vi "Read.vi"() -> ()   [LabVIEW 2013]
uses:
  <vilib>/NI/Modbus Library/API/Master/Modbus Master.lvclass
  <vilib>/NI/Modbus Library/API/Wrapper/Create TCP Master.vi
  GlobalStop.vi
  GlobalGraph.vi
  <vilib>/NI/Modbus Library/API/Wrapper/API Main.lvlib
panel:
  out "error out":errorcluster
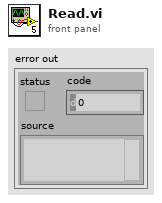
[diagram p1: front panel]
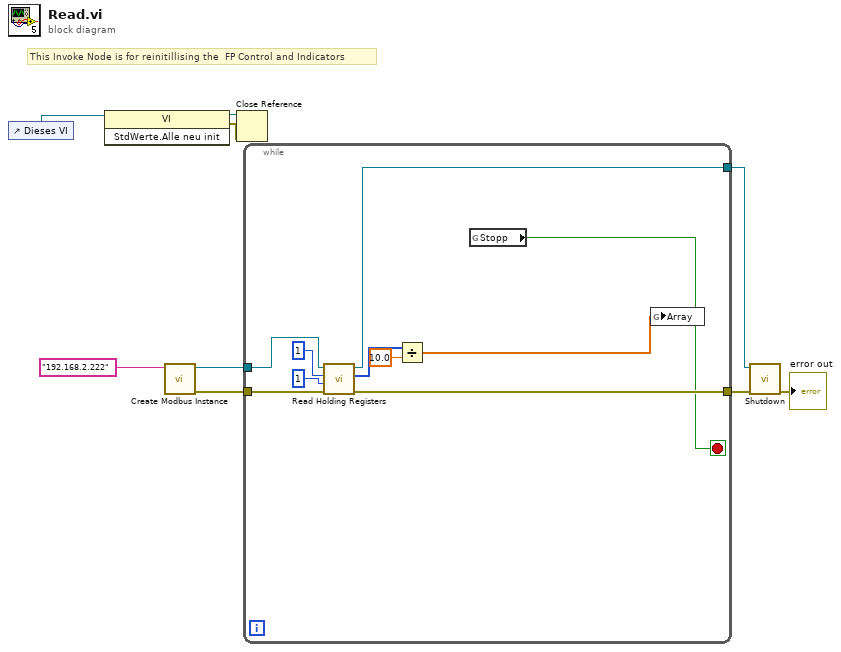
[diagram p0: block diagram]
diagram:
  # "This Invoke Node is for reinitillising the  FP Control and Indicators"
  n1 = control-ref of="Dieses VI"() -> (w3:refnum<vi>)
  n2 = invoke class="VI" method="StdWerte.Alle neu init"(reference=w3) -> (reference out=w2:refnum<vi>, error out=w1:errorcluster)  [unwired: 2 in, 1 out]
  n3 = call-poly <vilib>:"Create Modbus Instance.vi"("address"="192.168.2.222") -> ("error out"=w7:errorcluster, "TCP master instance"=w9:refnum<class "Modbus Master.lvclass">)  [unwired: 9 in]
  n4 = Close Reference(reference=w2, error in (no error)=w1) -> ()  [unwired: 1 out]
  n5 = while {
    tunnel: w9 -> [w19]
    tunnel: [w18] -> w8
    tunnel: w7 -> [w17]
    tunnel: [w16] -> w6
    stop <- w10 stop-if-true
    n6 = call-dynamic "Read Holding Registers.vi"("error in"=w17, "number of inputs"=u16 1, "starting address"=u16 1, "Modbus master in"=w19) -> ("error out"=w16:errorcluster, "register values"=w12:u16[], "Modbus master out"=w18:refnum<class "Modbus Master.lvclass">)  [unwired: 5 in]
    n7 = Divide(x=w12, y=10.0) -> (x/y=w11:dbl[])
    n8 = global read "GlobalStop.vi" "Stopp"() -> (w10:bool)
    n9 = global write "GlobalGraph.vi" "Array"(w11) -> ()
  }
  n10 = call-dynamic "Shutdown.vi"("error in"=w6, "Modbus master in"=w8) -> ("error out"=→"error out":errorcluster)  [unwired: 9 in]
